vi "Traversesetup.vi"() -> ()   [LabVIEW 2011]
uses:
  Anemometry/Anemometry Sub Vis/Gen Trav/Trav_mode.ctl
  Anemometry/Anemometry Sub Vis/Controls/Tunnel_Coordinates.ctl
  Anemometry/Anemometry Sub Vis/Controls/User_Specific_mode.ctl
  <vilib>/Utility/file.llb/Write To Spreadsheet File (DBL).vi
panel:
  in  "Loop Delay (s)":u32=15
  in  "Minimum Depth into soution (mm)":dbl=909.0
  in  "Number of Points Between Minimum and Maximum Depth":dbl=20.0
  in  "Maximum Depth into solution (mm)":dbl=1399.0
  in  "Save Location":path=path "C:/Documents and Settings/Adetola Elias/My Documents/Danial/Traverse Run.xls"
  in  "Sample Size for Density Meter Reading":i32=20
  in  "Delay For Density Meter Reading (s)":u32=15
  # "Time from Traverse to Density Meter = 14 Sec"
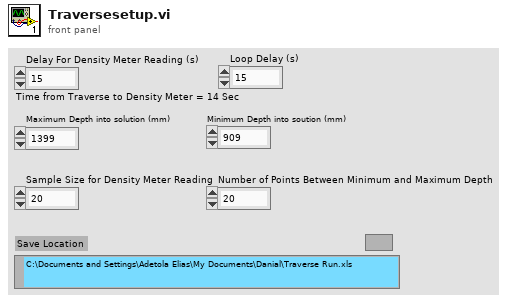
[diagram p1: front panel]
types:
  T1 = typedef "User_Specific_mode.ctl" = enum16{"Check VI only", "Run VI"}
  T2 = typedef "Tunnel_Coordinates.ctl" = enum16{"Work in Tunnel Coordinates", "Work in Model Coordinates"}
  T3 = typedef "Trav_mode.ctl" = enum16{"Move traverse", "Read traverse position", "Teach Position"}
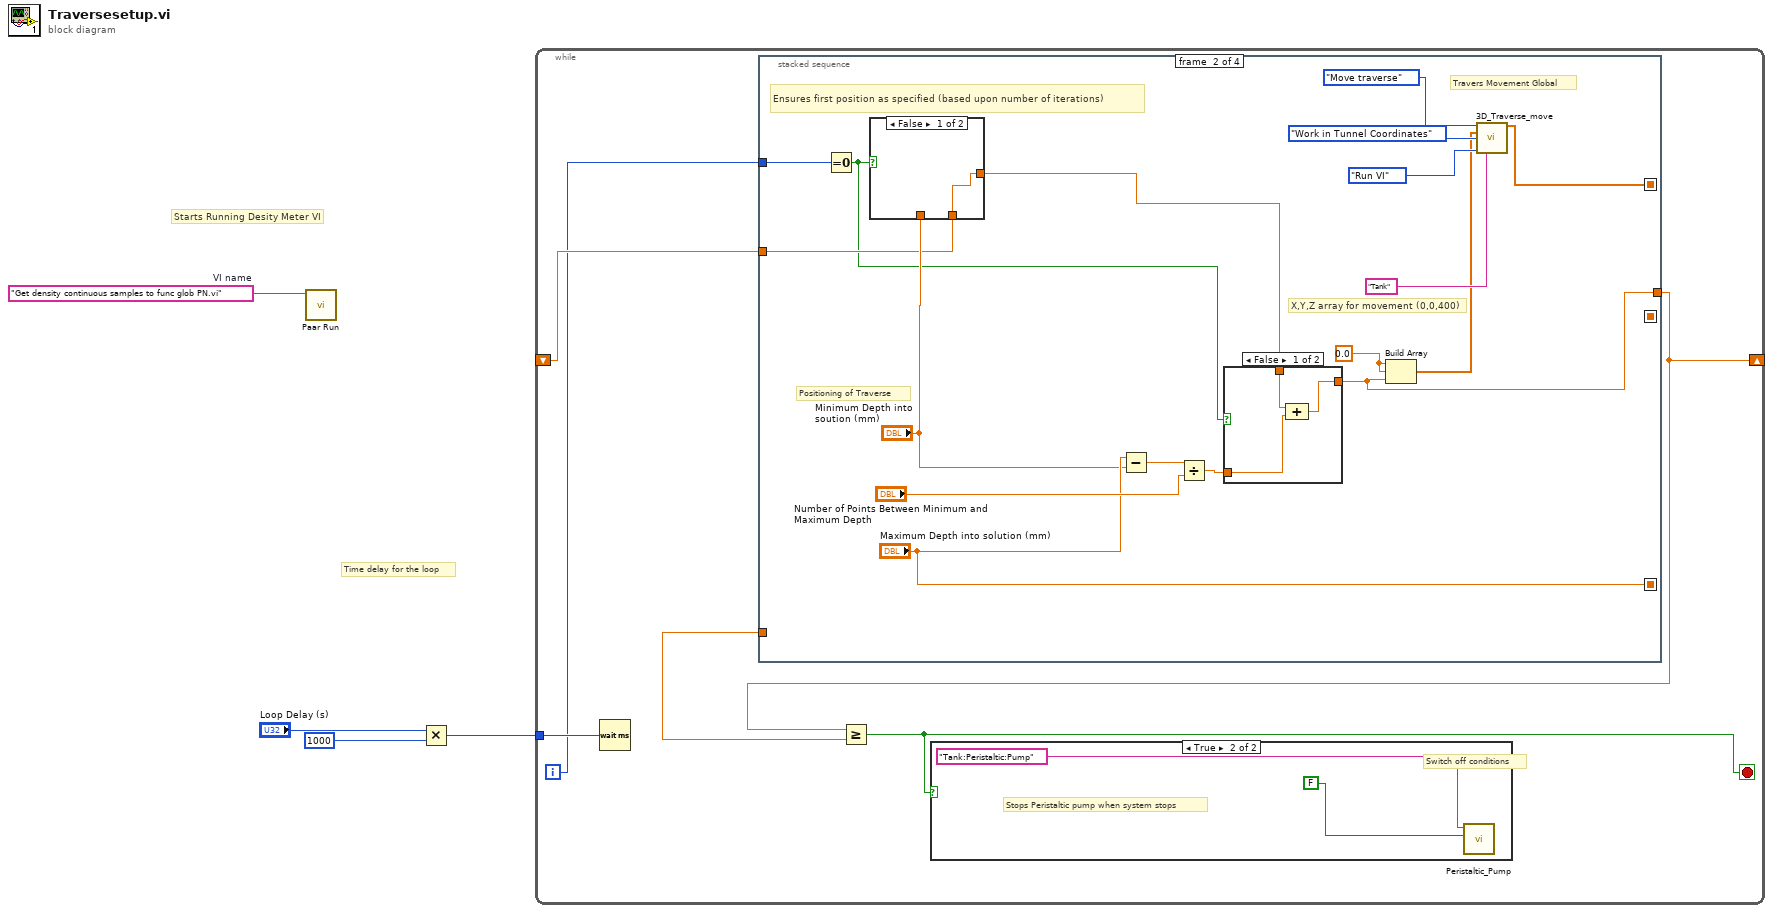
[diagram p0: block diagram]
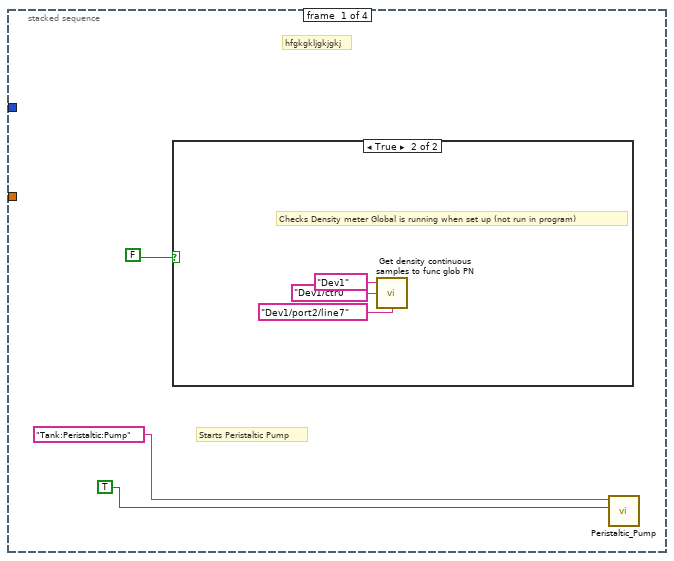
[diagram p3: hidden frame]
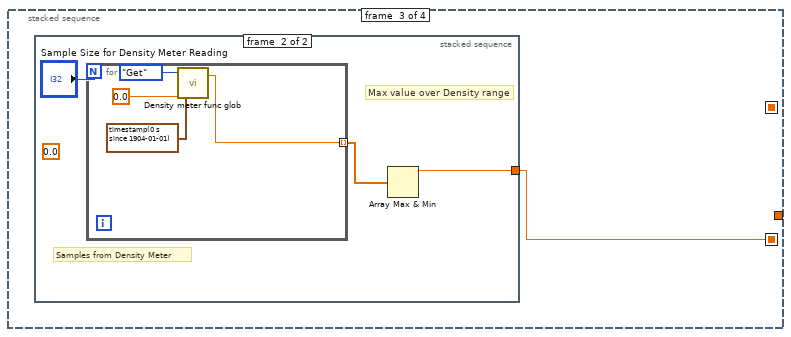
[diagram p7: hidden frame]
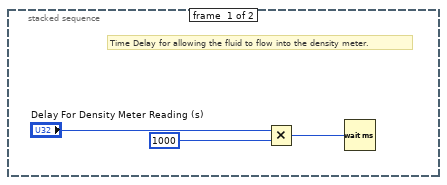
[diagram p8: hidden frame]
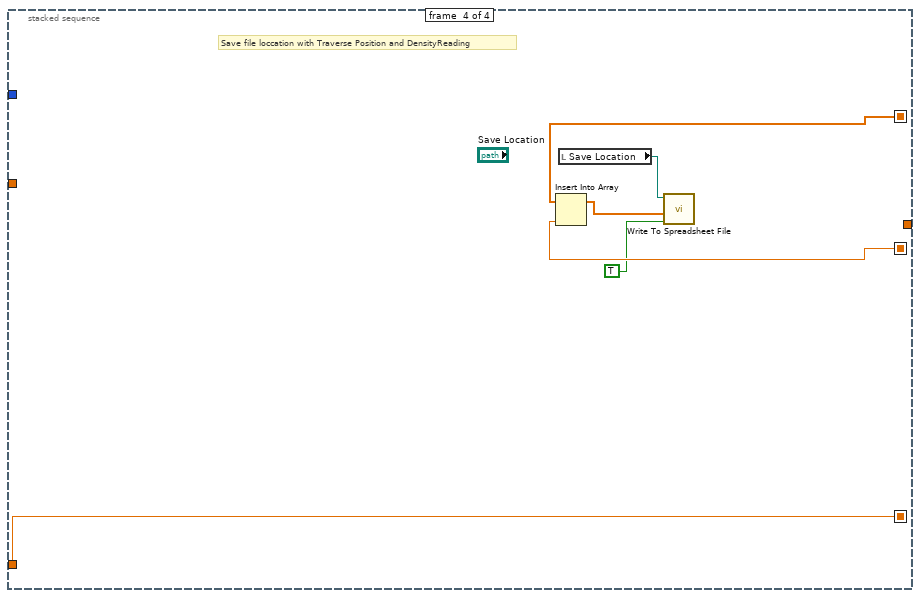
[diagram p9: hidden frame]
diagram:
  w3 = "Get density continuous samples to func glob PN.vi"  # VI name
  # "Time delay for the loop"
  # "Starts Running Desity Meter VI"
  n1 = call "Paar Run.vi"("VI name"=w3) -> ()  [unwired: 11 in]
  n2 = Multiply(x="Loop Delay (s)", y=1000 ("Sample Size 2")) -> (x*y=w4:u32)
  n3 = while {
    tunnel: w4 -> [w9]
    shift-right: [w8] -> _
    shift-left: _ -> [w7]
    i -> [w5]
    stop <- w6 stop-if-true
    # "Switch off conditions"
    n4 = Wait (ms)(milliseconds to wait=w9) -> ()  [unwired: 1 out]
    n5 = stacked-sequence {
      seq-local: [_ _ w42 _] -> [_ _ _ w56]
      seq-local: [_ w28 _ _] -> [_ _ _ w55]
      seq-local: [_ "Maximum Depth into solution (mm)" _ _] -> [_ _ _ w54]
      tunnel: w7 -> [_ w20 _ _]
      tunnel: [_ w29 _ _] -> w8
      tunnel: [_ _ _ w54] -> w10
      tunnel: w5 -> [_ w23 _ _]
      frame #0 {
        # "Starts Peristaltic Pump"
        # "hfgkgkljgkjgkj"
        n6 = case shown="True" FALSE {
          frame False {
          }
          frame True {
            # "Checks Density meter Global is running when set up (not run in program)"
            n7 = call "Get density continuous samples to func glob PN.vi"("Timing SW trigger"=tag "Dev1/port2/line7", "Counter"=tag "Dev1/ctr0", "Device"=tag "Dev1") -> ()
          }
        }
        n8 = call "Peristaltic_Pump.vi"("Boolean"=TRUE, "Channel Name"="Tank:Peristaltic:Pump") -> ()  [unwired: 8 in, 2 out]
      }
      frame #1 {
        w30 = 0.0 ("Density in")
        # "Positioning of Traverse"
        # "X,Y,Z array for movement (0,0,400)"
        # "Travers Movement Global"
        # "Ensures first position as specified (based upon number of iterations)"
        n9 = Equal To 0?(x=w23) -> (x = 0?=w19:bool)
        n10 = case shown="False" w19 {
          tunnel: [w36 w37] -> w21
          tunnel: "Minimum Depth into soution (mm)" -> [_ w37]
          tunnel: w20 -> [w36 _]
          frame False {
          }
          frame True {
          }
        }
        n11 = Subtract(x="Maximum Depth into solution (mm)", y="Minimum Depth into soution (mm)") -> (x-y=w27:dbl)
        n12 = Divide(x=w27, y="Number of Points Between Minimum and Maximum Depth") -> (x/y=w25:dbl)
        n13 = case shown="False" w19 {
          tunnel: w21 -> [w40 w41]
          tunnel: [w39 w41] -> w29
          tunnel: w25 -> [w38 _]
          frame False {
            n14 = Compound Arithmetic op=ADD(w40, w38) -> (w39:dbl)
          }
          frame True {
          }
        }
        n15 = Build Array(w30, w30, w29) -> (w31:dbl[])
        n16 = call "3D_Traverse_move.vi"("Mode"=Trav_mode."Move traverse", "Position"=w31, "Work in Tunnel Coordinates"=Tunnel_Coordinates."Work in Tunnel Coordinates", "Simulate/Run"=User_Specific_mode."Run VI", "Traverse name"="Tank") -> ("Trav Position achieved"=w28:dbl[])  [unwired: 8 in, 2 out]
      }
      frame #2 {
        n17 = stacked-sequence {
          tunnel: [_ w47] -> w42
          frame #0 {
            # "Time Delay for allowing the fluid to flow into the density meter."
            n18 = Multiply(x="Delay For Density Meter Reading (s)", y=1000 ("Sample Size 2")) -> (x*y=w44:u32)
            n19 = Wait (ms)(milliseconds to wait=w44) -> ()  [unwired: 1 out]
          }
          frame #1 {
            (unwired) 0.0 ("Actual Density (kg/m3) 2")
            # "Max value over Density range"
            # "Samples from Density Meter"
            n20 = for {
              N: "Sample Size for Density Meter Reading" -> [_]
              tunnel: [w49] -> w46 mode=indexing
              n21 = call "Density meter func glob.vi"("Sample DateTime in"=timestamp(0 s since 1904-01-01), "Density in"=0.0, "Action"=enum16{"Get", "Set"}."Get") -> ("Density out"=w49:dbl)  [unwired: 1 out]
            }
            n22 = Array Max & Min(array=w46) -> (max value=w47:dbl)  [unwired: 3 out]
          }
        }
      }
      frame #3 {
        # "Save file loccation with Traverse Position and DensityReading"
        n23 = Insert Into Array(array=w55, new element=w56) -> (w57:dbl[])  [unwired: 1 in]
        n24 = local read "Save Location"() -> (w58:path)
        n25 = call-poly <vilib>:"Write To Spreadsheet File.vi"("append to file? (new file:F)"=TRUE, "1D data"=w57, "file path (dialog if empty)"=w58) -> ()  [unwired: 5 in, 1 out]
      }
    }
    n26 = Greater Or Equal?(x=w8, y=w10) -> (x >= y?=w6:bool)
    n27 = case shown="True" w6 {
      frame False {
      }
      frame True {
        # "Stops Peristaltic pump when system stops"
        n28 = call "Peristaltic_Pump.vi"("Boolean"=FALSE, "Channel Name"="Tank:Peristaltic:Pump") -> ()  [unwired: 8 in, 2 out]
      }
    }
  }
